vi "ActiveObject_QueueQueue_ProcessRepository_Native.vi"(0 "reference in":refnum<class>, 1 "Action(ReadRepository)":T1(ring), 5 "error in (no error)":errorcluster) -> (9 "ProcessViRef":refnum<vi>, 11 "ProcessSyncQueue":refnum<queue>, 13 "FromProcessQueue":refnum<queue>, 14 "reference out":refnum<class>, 15 "ToProcessQueue":refnum<queue>, 17 "ProcessAlreadyStarted":bool, 19 "error out":errorcluster)   [LabVIEW 2012]
uses:
  <resource>/Framework/Providers/Open_GDS/ClassProviders/DesignPatterns/ActiveObjects/ActiveObjects_QueueQueue_SubVIs/ActiveObject_QueueQueue_Process.ctl
panel:
  # "Use this indicator for sending messages to the Process VI"
  # "These indicators are used by the process VIs"
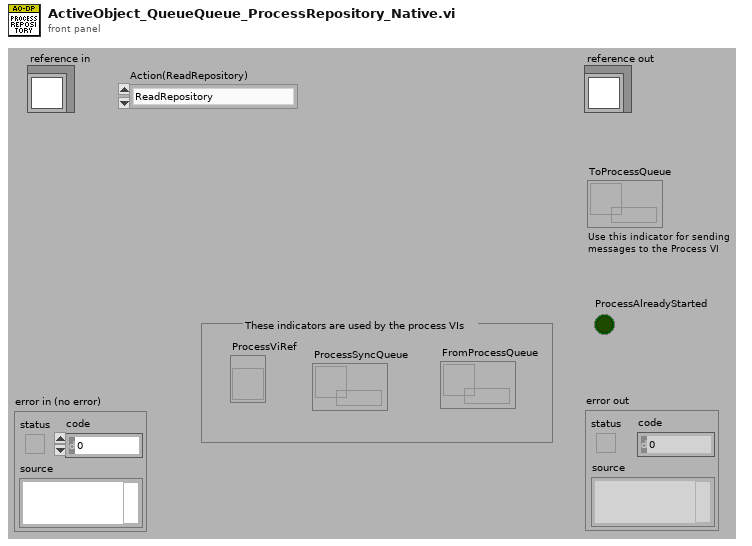
[diagram p1: front panel]
types:
  T1 = enum16{"ReadRepository", "CreateNew", "CreateOrLookUpExisting", "ReadRepositoryAndDestroy"}
  T2 = typedef "ActiveObject_QueueQueue_Process.ctl" = cluster{"ToProcessQueue":refnum<queue>, "FromProcessQueue":refnum<queue>, "ProcessSyncQueue":refnum<queue>, "ProcessViRef":refnum<vi>}
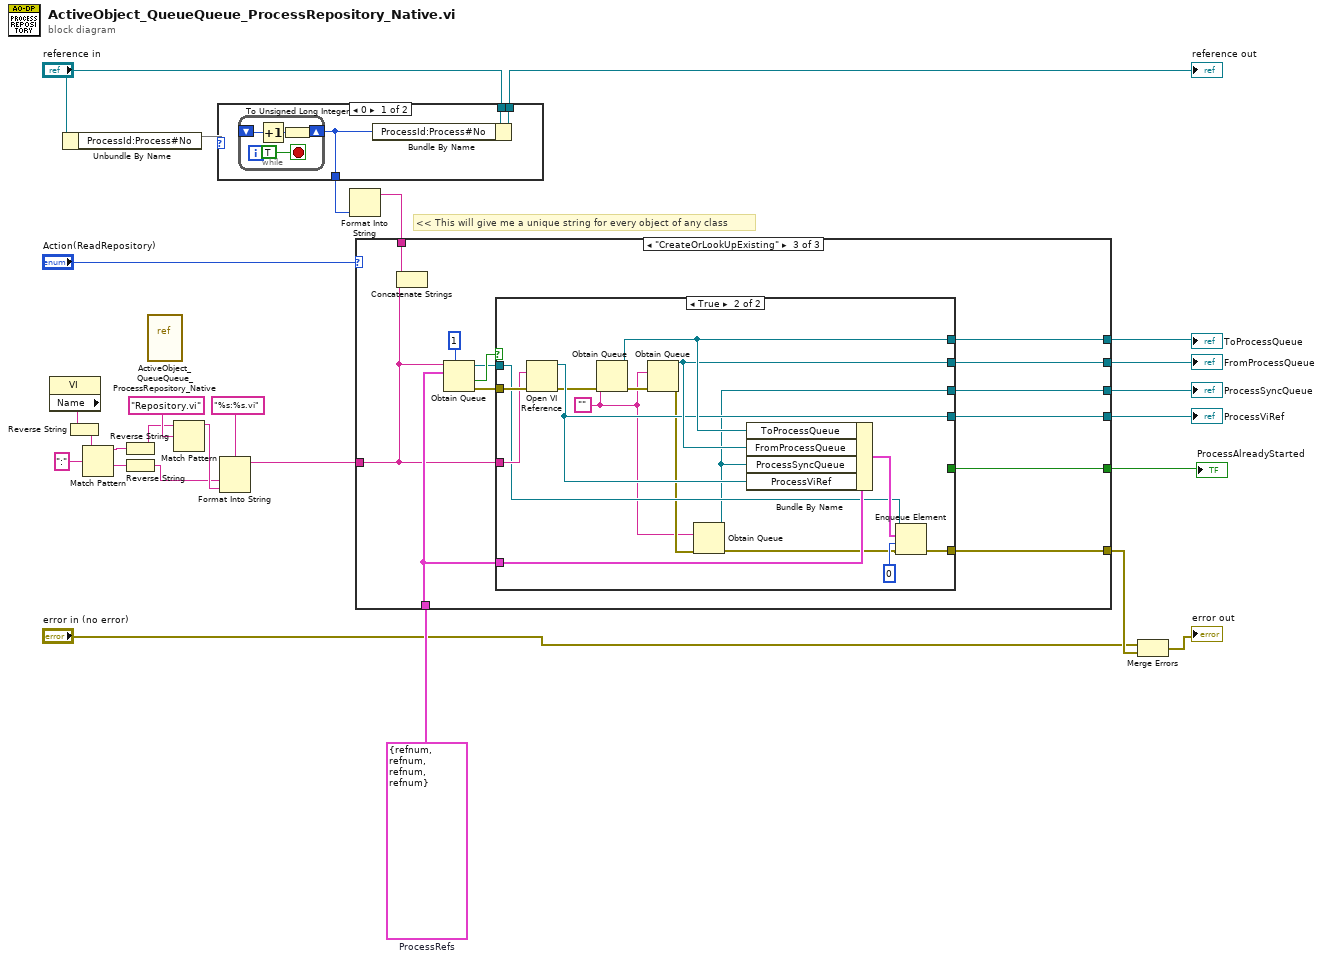
[diagram p0: block diagram]
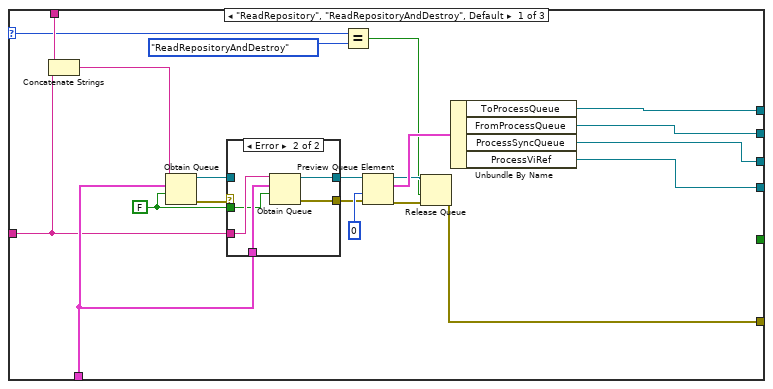
[diagram p3: hidden frame]
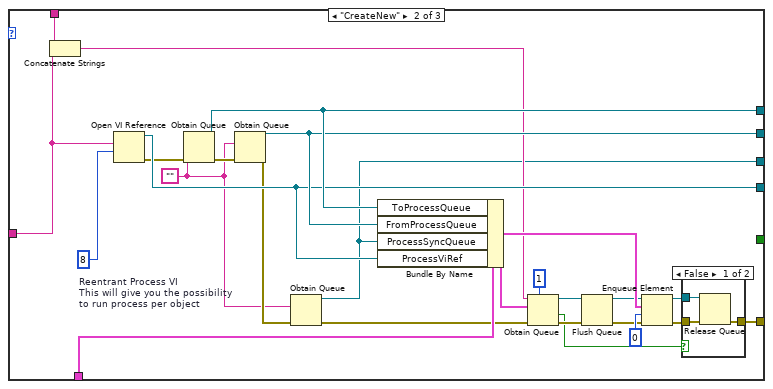
[diagram p5: hidden frame]
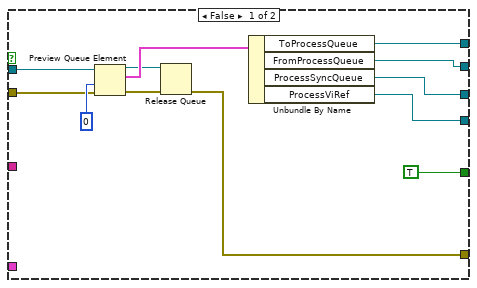
[diagram p7: hidden frame]
diagram:
  w21 = T2 {"ToProcessQueue"=refnum, "FromProcessQueue"=refnum, "ProcessSyncQueue"=refnum, "ProcessViRef"=refnum}  # ProcessRefs
  # "<< This will give me a unique string for every object of any class"
  n1 = property class="VI"() -> ("Name"=w10:string)  [unwired: 2 in, 2 out]
  n2 = Unbundle By Name("reference in") -> ("ProcessId:Process#No"=w4)
  n3 = Reverse String(1:w10) -> (0:w11:string)
  n4 = Match Pattern(string=w11, regular expression=":") -> (before substring=w15:string, after substring=w12:string)  [unwired: 1 in, 2 out]
  n5 = Reverse String(1:w15) -> (0:w16:string)
  n6 = Reverse String(1:w12) -> (0:w14:string)
  n7 = vi-ref <resource>:"ActiveObject_QueueQueue_ProcessRepository_Native.vi"() -> ()  [unwired: 1 out]
  n8 = Match Pattern(string=w16, regular expression="Repository.vi") -> (before substring=w18:string)  [unwired: 1 in, 3 out]
  n9 = case shown="0" w4 {
    selector: w4 -> [_ w35]
    tunnel: [w27 w35] -> w5
    tunnel: "reference in" -> [w29 w34]
    tunnel: [w28 w34] -> w2
    frame 0 {
      n10 = while {
        shift-right: [w30] -> w27
        shift-left: _ -> [w32]
        stop <- TRUE stop-if-true
        n11 = Increment(x=w32) -> (x+1=w31:u32)
        n12 = To Unsigned Long Integer(number=w31) -> (unsigned 32bit integer=w30:u32)
      }
      n13 = Bundle By Name(cluster=w29, "ProcessId:Process#No"=w27) -> (w28:refnum<class>)
    }
    frame Default {
    }
  }
  "reference out" <- w2
  n14 = Format Into String(format string="%s:%s.vi", w14, w18) -> (resulting string=w8:string)  [unwired: 2 in, 1 out]
  n15 = Format Into String(w5) -> (resulting string=w1:string)  [unwired: 3 in, 1 out]
  n16 = case shown="\"CreateOrLookUpExisting\"" "Action(ReadRepository)" {
    selector: "Action(ReadRepository)" -> [w38 _ _]
    tunnel: [w51 w71 w103] -> w25
    tunnel: [w53 w88 w105] -> w23
    tunnel: [w52 w87 w104] -> w24
    tunnel: [w54 w86 w102] -> w22
    tunnel: w21 -> [w46 w78 w98]
    tunnel: w1 -> [w44 w77 w94]
    tunnel: [w39 w65 w101] -> w19
    tunnel: w8 -> [w43 w75 w93]
    tunnel: [_ _ w96] -> w7
    frame "ReadRepository", "ReadRepositoryAndDestroy", Default {
      w45 = FALSE ("create if not found? (T)")
      n17 = Concatenate Strings(w44, w43) -> (w42:string)
      n18 = Obtain Queue(name (unnamed)=w42, element data type=w46, create if not found? (T)=w45) -> (queue out=w48:refnum<queue>, error out=w50:errorcluster)  [unwired: 2 in, 1 out]
      n19 = case shown="Error" w50 {
        selector: w50 -> [w58 _]
        tunnel: [w58 w60] -> w49
        tunnel: w48 -> [w57 _]
        tunnel: [w57 w61] -> w47
        tunnel: w46 -> [_ w63]
        tunnel: w43 -> [_ w62]
        tunnel: w45 -> [_ w59]
        frame No Error {
        }
        frame Error {
          n20 = Obtain Queue(name (unnamed)=w62, element data type=w63, create if not found? (T)=w59) -> (queue out=w61:refnum<queue>, error out=w60:errorcluster)  [unwired: 2 in, 1 out]
        }
      }
      n21 = Equal?(x=w38, y=T1."ReadRepositoryAndDestroy") -> (x = y?=w37:bool)
      n22 = Preview Queue Element(queue=w47, timeout in ms (-1)=0, error in (no error)=w49) -> (queue out=w41:refnum<queue>, element=w55:T2, error out=w40:errorcluster)  [unwired: 1 out]
      n23 = Release Queue(queue=w41, force destroy? (F)=w37, error in (no error)=w40) -> (error out=w39:errorcluster)  [unwired: 2 out]
      n24 = Unbundle By Name(w55) -> ("ToProcessQueue"=w53:refnum<queue>, "FromProcessQueue"=w52:refnum<queue>, "ProcessSyncQueue"=w51:refnum<queue>, "ProcessViRef"=w54:refnum<vi>)
    }
    frame "CreateNew" {
      w83 = 8  # Reentrant Process VI This will give you the possibility to run process per object
      w72 = ""
      n25 = Concatenate Strings(w77, w75) -> (w76:string)
      n26 = Open VI Reference(vi path=w75, options=w83) -> (vi reference=w86:refnum<vi>, error out=w84:errorcluster)  [unwired: 4 in]
      n27 = Obtain Queue(element data type=w72, error in (no error)=w84) -> (queue out=w88:refnum<queue>, error out=w85:errorcluster)  [unwired: 3 in, 1 out]
      n28 = Obtain Queue(element data type=w72, error in (no error)=w85) -> (queue out=w87:refnum<queue>, error out=w74:errorcluster)  [unwired: 3 in, 1 out]
      n29 = Obtain Queue(element data type=w72, error in (no error)=w74) -> (queue out=w71:refnum<queue>, error out=w73:errorcluster)  [unwired: 3 in, 1 out]
      n30 = Bundle By Name(cluster=w78, "ToProcessQueue"=w88, "FromProcessQueue"=w87, "ProcessSyncQueue"=w71, "ProcessViRef"=w86) -> (w81:T2)
      n31 = Obtain Queue(max queue size (-1, unlimited)=1, name (unnamed)=w76, element data type=w81, error in (no error)=w73) -> (queue out=w82:refnum<queue>, created new?=w64:bool, error out=w69:errorcluster)  [unwired: 1 in]
      n32 = Flush Queue(queue=w82, error in (no error)=w69) -> (queue out=w70:refnum<queue>, error out=w68:errorcluster)  [unwired: 1 out]
      n33 = Enqueue Element(queue=w70, element=w81, timeout in ms (-1)=0, error in (no error)=w68) -> (queue out=w66:refnum<queue>, error out=w67:errorcluster)  [unwired: 1 out]
      n34 = case shown="False" w64 {
        tunnel: w67 -> [w91 w92]
        tunnel: w66 -> [w90 _]
        tunnel: [w89 w92] -> w65
        frame False {
          n35 = Release Queue(queue=w90, error in (no error)=w91) -> (error out=w89:errorcluster)  [unwired: 1 in, 2 out]
        }
        frame True {
        }
      }
    }
    frame "CreateOrLookUpExisting" {
      n36 = Concatenate Strings(w94, w93) -> ()  [unwired: 1 out]
      n37 = Obtain Queue(max queue size (-1, unlimited)=1, name (unnamed)=w93, element data type=w98) -> (queue out=w99:refnum<queue>, created new?=w100:bool, error out=w97:errorcluster)  [unwired: 2 in]
      n38 = case shown="True" w100 {
        tunnel: [w117 w133] -> w105
        tunnel: [w116 w132] -> w104
        tunnel: [w115 w118] -> w103
        tunnel: [w114 w131] -> w102
        tunnel: [w107 w130] -> w101
        tunnel: w98 -> [_ w129]
        tunnel: w97 -> [w111 w124]
        tunnel: w93 -> [_ w123]
        tunnel: w99 -> [w112 w122]
        tunnel: [TRUE _] -> w96
        frame False {
          n39 = Preview Queue Element(queue=w112, timeout in ms (-1)=0, error in (no error)=w111) -> (queue out=w106:refnum<queue>, element=w110:T2, error out=w108:errorcluster)  [unwired: 1 out]
          n40 = Release Queue(queue=w106, error in (no error)=w108) -> (error out=w107:errorcluster)  [unwired: 1 in, 2 out]
          n41 = Unbundle By Name(w110) -> ("ToProcessQueue"=w117:refnum<queue>, "FromProcessQueue"=w116:refnum<queue>, "ProcessSyncQueue"=w115:refnum<queue>, "ProcessViRef"=w114:refnum<vi>)
        }
        frame True {
          w119 = ""
          n42 = Open VI Reference(vi path=w123, error in (no error)=w124) -> (vi reference=w131:refnum<vi>, error out=w127:errorcluster)  [unwired: 4 in]
          n43 = Obtain Queue(element data type=w119, error in (no error)=w127) -> (queue out=w133:refnum<queue>, error out=w128:errorcluster)  [unwired: 3 in, 1 out]
          n44 = Obtain Queue(element data type=w119, error in (no error)=w128) -> (queue out=w132:refnum<queue>, error out=w121:errorcluster)  [unwired: 3 in, 1 out]
          n45 = Obtain Queue(element data type=w119, error in (no error)=w121) -> (queue out=w118:refnum<queue>, error out=w120:errorcluster)  [unwired: 3 in, 1 out]
          n46 = Bundle By Name(cluster=w129, "ToProcessQueue"=w133, "FromProcessQueue"=w132, "ProcessSyncQueue"=w118, "ProcessViRef"=w131) -> (w126:T2)
          n47 = Enqueue Element(queue=w122, element=w126, timeout in ms (-1)=0, error in (no error)=w120) -> (error out=w130:errorcluster)  [unwired: 2 out]
        }
      }
    }
  }
  "ProcessSyncQueue" <- w25
  "ToProcessQueue" <- w23
  "FromProcessQueue" <- w24
  "ProcessViRef" <- w22
  "ProcessAlreadyStarted" <- w7
  n48 = Merge Errors("error in (no error)", w19) -> (→"error out":errorcluster)
